vi "2.9.vi"() -> ()   [LabVIEW 2017]
panel:
  in  "Color Box":u32(colorbox)
  out "Waveform Chart":dbl(graph)
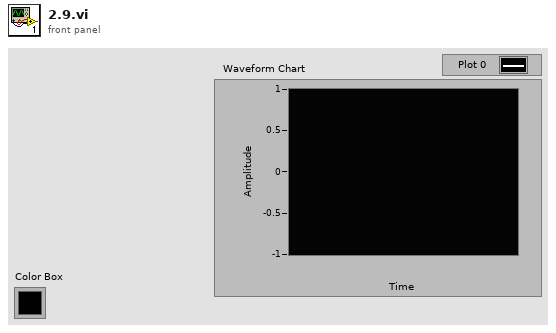
[diagram p1: front panel]
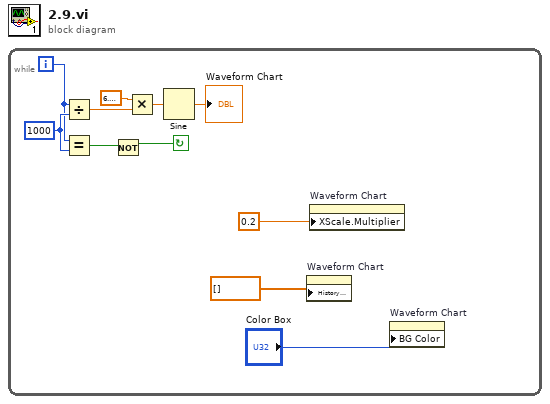
[diagram p0: block diagram]
diagram:
  n1 = while {
    i -> [w9]
    stop <- w5 continue-if-true
    w10 = 1000
    n2 = Divide(x=w9, y=w10) -> (x/y=w8:dbl)
    n3 = Equal?(x=w9, y=w10) -> (x = y?=w4:bool)
    n4 = Not(x=w4) -> (.not. x?=w5:bool)
    n5 = Multiply(x=6.283185307179586, y=w8) -> (x*y=w7:dbl)
    n6 = Sine(x=w7) -> (sin(x)=→"Waveform Chart":dbl)
    n7 = property on="Waveform Chart" class="WFChart (strict)"("History Data"=dbl[] []) -> ()  [unwired: 2 in, 2 out]
    n8 = property on="Waveform Chart" class="WFChart (strict)"("XScale.Multiplier"=0.2) -> ()  [unwired: 2 in, 2 out]
    n9 = property on="Waveform Chart" class="WFChart (strict)"("BG Color"="Color Box") -> ()  [unwired: 2 in, 2 out]
  }
